vi "Cairo.OpenConnectionFromFile.vi"(11 "File Path":path) -> (0 "Error Out":errorcluster, 3 "Refnum":T1)   [LabVIEW 2019]
uses:
  <vilib>/Utility/config.llb/Config Data RefNum.ctl
  <vilib>/Utility/config.llb/NI_LVConfig.lvlib
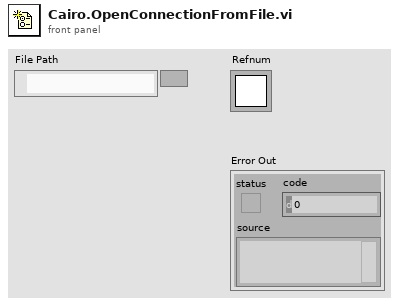
[diagram p1: front panel]
types:
  T1 = typedef "NI_LVConfig.lvlib/Config Data RefNum.ctl" = refnum<k1>
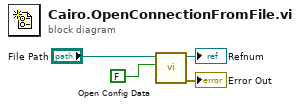
[diagram p0: block diagram]
diagram:
  n1 = call <vilib>:"Open Config Data.vi"("create file if necessary (T)"=FALSE, "configuration file path"="File Path") -> ("error out"=→"Error Out":errorcluster, "refnum"=→"Refnum":T1)  [unwired: 7 in, 1 out]
